vi "send_shifted_influent.vi"(4 "State":i16, 5 "Time":dbl format="%.2f", 6 "Sensor Values":dbl[](array[numeric]), 7 "Set Points":dbl[](array[numeric])) -> (0 "required data":T1={"Set Point names"=["", ""], "required number of setpoints"=0, "required number of sensors"=0, "Sensor names"=["sensor 1"]}, 3 "output value":dbl)   [LabVIEW 2019]
uses:
  store_last_RowData.vi
panel:
  # "Enter the correct information for this control code in the required data structure below. Then make the current value default by right clicking on the border of the data structure. Select \"data operations\" and then select \"make current value default\". These values will be displayed by process controller."
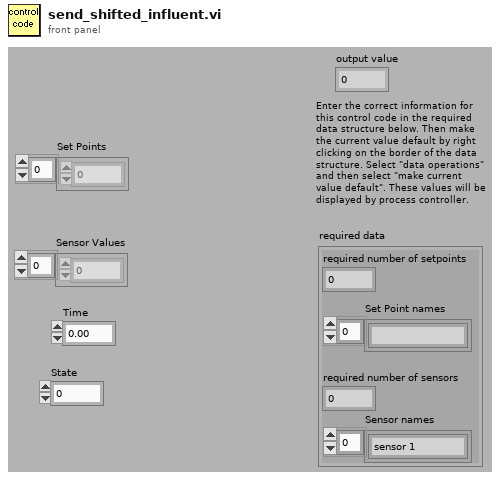
[diagram p1: front panel]
types:
  T1 = cluster{"Set Point names":string[], "required number of setpoints":u8, "required number of sensors":u8, "Sensor names":string[]}
  T2 = typedef "RowData_Type.ctl" = cluster{"C_raw(mg/L)":dbl, "C_clarified(mg/L)":dbl, "C_floc(mg/L)":dbl, "floc_sat":dbl, "C_DOM":dbl, "C_coag(mg/L)":dbl, "C_clar_target(mg/L)":dbl}
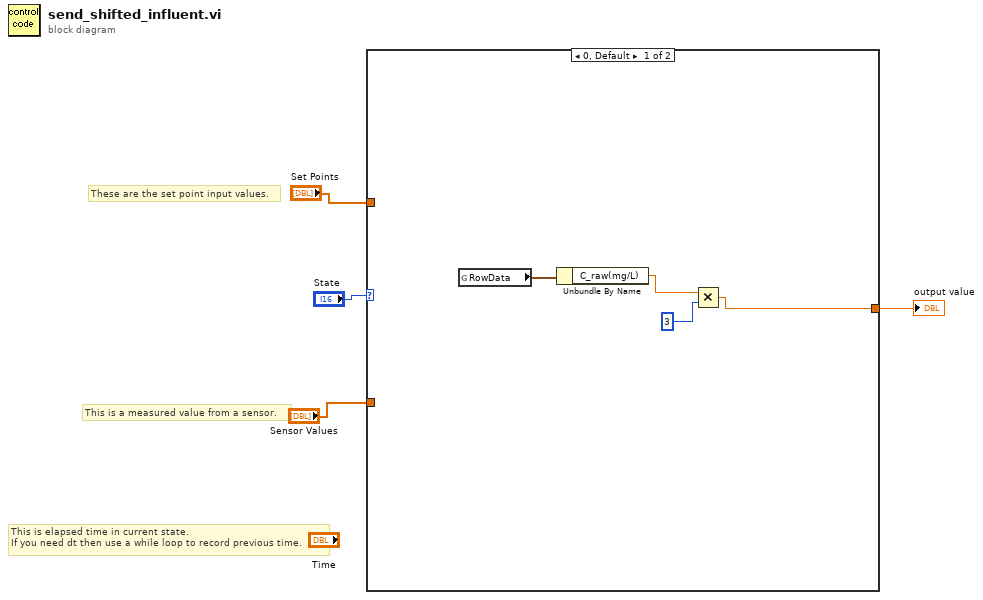
[diagram p0: block diagram]
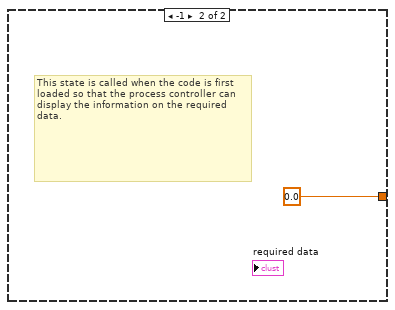
[diagram p2: hidden frame]
diagram:
  # "These are the set point input values."
  # "This is a measured value from a sensor."
  # "This is elapsed time in current state.\nIf you need dt then use a while loop to record previous time."
  n1 = case shown="0, Default" "State" {
    tunnel: [w5 0.0 ("fraction on")] -> w3
    tunnel: "Set Points" -> [_ _]
    tunnel: "Sensor Values" -> [_ _]
    frame 0, Default {
      n2 = global read "store_last_RowData.vi" "RowData"() -> (w8:T2)
      n3 = Unbundle By Name(w8) -> ("C_raw(mg/L)"=w7:dbl)
      n4 = Multiply(x=w7, y=3) -> (x*y=w5:dbl)
    }
    frame -1 {
      # "This state is called when the code is first loaded so that the process controller can display the information on the required data."
    }
  }
  "output value" <- w3
